vi "Obtain Message Queue.vi"(8 "error in (no error)":errorcluster, 11 "PID Loop in":refnum<class "PID Loop.lvclass">) -> (0 "error out":errorcluster, 3 "PID Loop out":refnum<class "PID Loop.lvclass">)   [LabVIEW 2024, in "PID Loop.lvlib" / "PID Loop.lvclass"]
uses:
  PID Loop.lvclass
  PID Loop.lvclass/PID Loop.ctl
  Message.ctl
  Messages.ctl
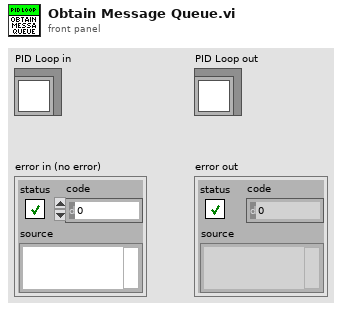
[diagram p1: front panel]
types:
  T1 = typedef "PID Loop.lvlib/PID Loop.lvclass/Message.ctl" = cluster{"Message":T2, "Data":variant}
  T2 = typedef "PID Loop.lvlib/PID Loop.lvclass/Messages.ctl" = enum16{"Stop", "Start", "Exit", "Poll"}
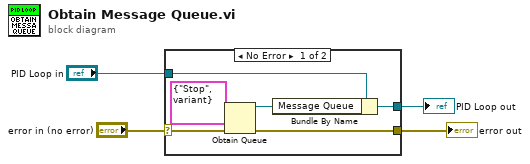
[diagram p0: block diagram]
diagram:
  n1 = case shown="No Error" "error in (no error)" {
    selector: "error in (no error)" -> [w7 w12]
    tunnel: [w6 w12] -> w3
    tunnel: [w5 w11] -> w1
    tunnel: "PID Loop in" -> [w9 w11]
    frame No Error {
      n2 = Obtain Queue(element data type=T1 {"Message"=enum."Stop", "Data"=variant} ("Message"), error in (no error)=w7) -> (queue out=w8:refnum<queue>, error out=w6:errorcluster)  [unwired: 3 in, 1 out]
      n3 = Bundle By Name(cluster=w9, "Message Queue"=w8) -> (w5:refnum<class "PID Loop.lvclass">)
    }
    frame Error {
    }
  }
  "error out" <- w3
  "PID Loop out" <- w1
